vi "ITC 503 -- set gas flow.vi"(8 "error in":errorcluster, 10 "Gas %":dbl, 11 "ITC503 Address":refnum<visa-resource-name>="GPIB0::24::INSTR") -> (0 "error out":errorcluster, 3 "ITC503 Address OUT":refnum<visa-resource-name>="GPIB0::24::INSTR")   [LabVIEW 2010]
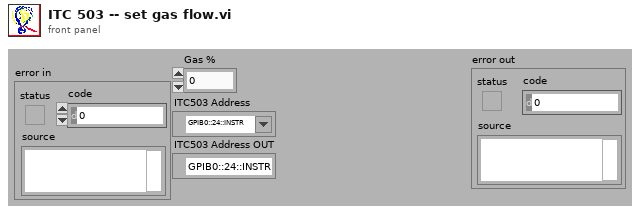
[diagram p1: front panel]
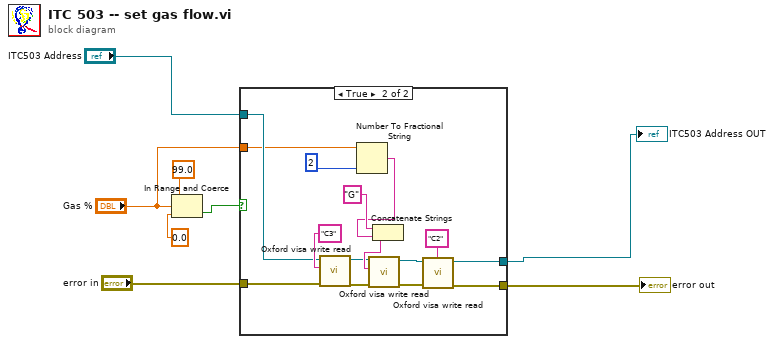
[diagram p0: block diagram]
diagram:
  n1 = In Range and Coerce(upper limit=99.0, x="Gas %", lower limit=0.0) -> (In Range?=w5:bool)  [unwired: 1 out]
  n2 = case shown="True" w5 {
    tunnel: "error in" -> [w10 w17]
    tunnel: [w10 w16] -> w4
    tunnel: "ITC503 Address" -> [w9 w15]
    tunnel: [w9 w12] -> w2
    tunnel: "Gas %" -> [_ w11]
    frame False {
      # "need to rize some kind of error ..."
    }
    frame True {
      n3 = call "Oxford visa write read.vi"("error in (no error)"=w17, "write buffer"="C3" ("Command"), "VISA resource name"=w15) -> ("error out"=w21:errorcluster, "VISA resource name out"=w14:refnum<visa-resource-name>)  [unwired: 6 in, 1 out]
      n4 = Number To Fractional String(number=w11, precision (6)=i16 2) -> (F-format string=w22:string)  [unwired: 2 in]
      n5 = Concatenate Strings("G" ("string"), w22) -> (w19:string)
      n6 = call "Oxford visa write read.vi"("error in (no error)"=w21, "write buffer"=w19, "VISA resource name"=w14) -> ("error out"=w20:errorcluster, "VISA resource name out"=w13:refnum<visa-resource-name>)  [unwired: 6 in, 1 out]
      n7 = call "Oxford visa write read.vi"("error in (no error)"=w20, "write buffer"="C2" ("Command"), "VISA resource name"=w13) -> ("error out"=w16:errorcluster, "VISA resource name out"=w12:refnum<visa-resource-name>)  [unwired: 6 in, 1 out]
    }
  }
  "error out" <- w4
  "ITC503 Address OUT" <- w2
